vi "path_db.vi"(8 "error in":errorcluster) -> (0 "error out":errorcluster, 3 "resulting string":path)   [LabVIEW 2017]
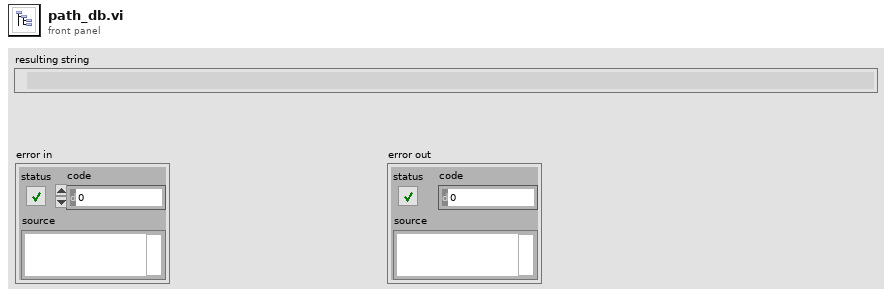
[diagram p1: front panel]
types:
  T1 = enum32{"invalid app kind", "Development System", "Run Time System", "Student Edition", "Embedded LabVIEW", "Evaluation", "Custom"}
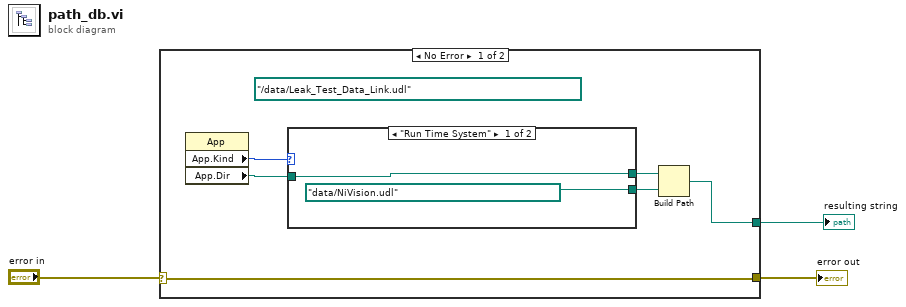
[diagram p0: block diagram]
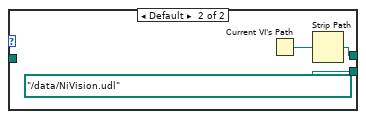
[diagram p2: hidden frame]
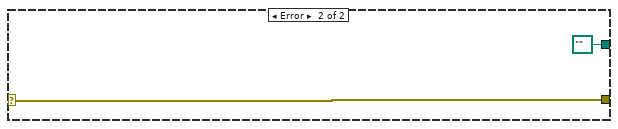
[diagram p3: hidden frame]
diagram:
  n1 = case shown="No Error" "error in" {
    selector: "error in" -> [w5 w16]
    tunnel: [w4 path "" ("appended path")] -> w3
    tunnel: [w5 w16] -> w1
    frame No Error {
      (unwired) path "../data/Leak_Test_Data_Link.udl" ("path")
      n2 = property class="App"() -> ("App.Kind"=w9:T1, "App.Dir"=w8:path)  [unwired: 2 in, 2 out]
      n3 = case shown="\"Run Time System\"" w9 {
        tunnel: w8 -> [w11 _]
        tunnel: [path "data/NiVision.udl" ("path") path "../data/NiVision.udl" ("path")] -> w7
        tunnel: [w11 w12] -> w6
        frame "Run Time System" {
        }
        frame Default {
          n4 = Current VI's Path() -> (path=w13:path)
          n5 = Strip Path(path=w13) -> (stripped path=w12:path)  [unwired: 1 out]
        }
      }
      n6 = Build Path(base path=w6, name or relative path=w7) -> (appended path=w4:path)
    }
    frame Error {
    }
  }
  "resulting string" <- w3
  "error out" <- w1
